vi "waveform.vi"() -> ()   [LabVIEW 2017]
panel:
  in  "t0 2":timestamp
  out "Waveform Graph":dynamicdata(graph)
  in  "dt":dbl
  in  "t0":timestamp
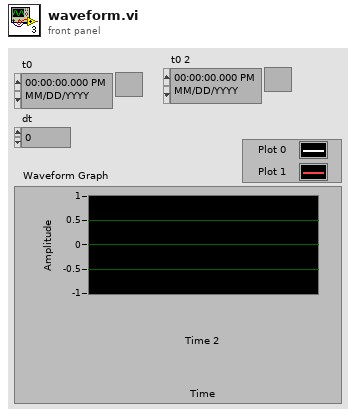
[diagram p1: front panel]
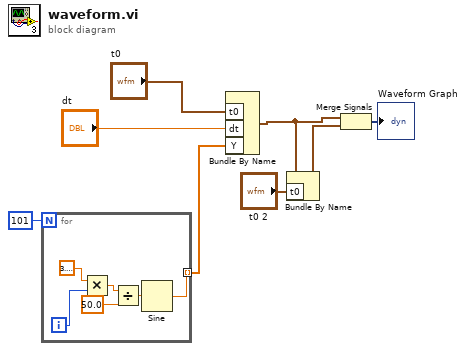
[diagram p0: block diagram]
diagram:
  n1 = for {
    N: 101 -> [_]
    tunnel: [w9] -> w5 mode=indexing
    i -> [w10]
    n2 = Multiply(x=3.141592653589793, y=w10) -> (x*y=w14:dbl)
    n3 = Divide(x=w14, y=50.0) -> (x/y=w13:dbl)
    n4 = Sine(x=w13) -> (sin(x)=w9:dbl)
  }
  n5 = Bundle By Name("t0"="t0", "dt"="dt", "Y"=w5) -> (w4:waveform(dbl))  [unwired: 1 in]
  n6 = Bundle By Name(cluster=w4, "t0"="t0 2") -> (w3:waveform(dbl))
  n7 = Merge Signals(w4, w3) -> (→"Waveform Graph":dynamicdata)
